vi "SDCP SMF Receiver and Transmitter - Transmit using data fromTx Table.vi"(3 "error in (no error)":errorcluster, 5 "Table Control":refnum<vi>) -> (0 "error out":errorcluster)   [LabVIEW 2020]
uses:
  Typedefs/SDCP SMF Receiver and Transmitter - Transmit Table Element.ctl
  Typedefs/SDCP SMF logger - SMF with timestamp.ctl
panel:
  out "Update table":bool
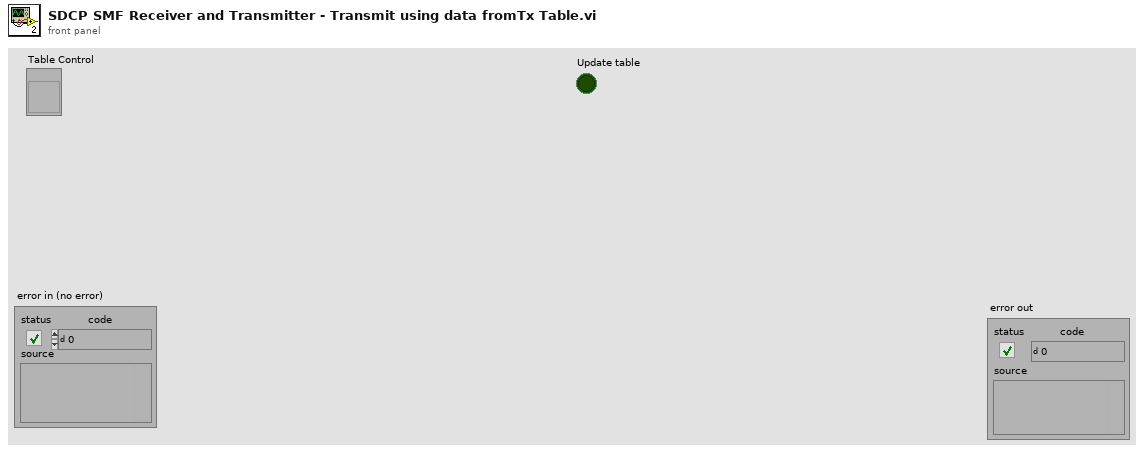
[diagram p1: front panel]
types:
  T1 = typedef "SDCP SMF Receiver and Transmitter - Transmit Table Element.ctl" = cluster{"Frame ID":i32, "Frame Name":string, "Data Bytes":u8[], "Cycle time (ms)":i32, "Counter":i32, "Trigger mode":enum16{"Triggered", "Cyclic"}, "Trigger state":enum16{"Stop cyclic trigger", "Start cyclic trigger", "Stop single trigger", "Start single trigger"}, "Parameter names":string[], "Parameter values":string[]}
  T2 = typedef "SDCP SMF Receiver and Transmitter - Notifier and Queues.ctl" = cluster{"Trace Queue":refnum<queue>, "Tx - Log Table Queue":refnum<queue>, "Tx - User Queue":refnum<queue>, "Rx - Log Table Queue":refnum<queue>, "Rx - User Queue":refnum<queue>, "Log status Notifier":refnum<notifier>, "Plot Queue":refnum<queue>}
  T3 = enum16{"Stop cyclic trigger", "Start cyclic trigger", "Stop single trigger", "Start single trigger"}
  T4 = typedef "SDCP SMF logger - SMF with timestamp.ctl" = cluster{"Bytes":u8[], "Checksum":bool, "Time (ms)":u32, "Tx/Rx":string}
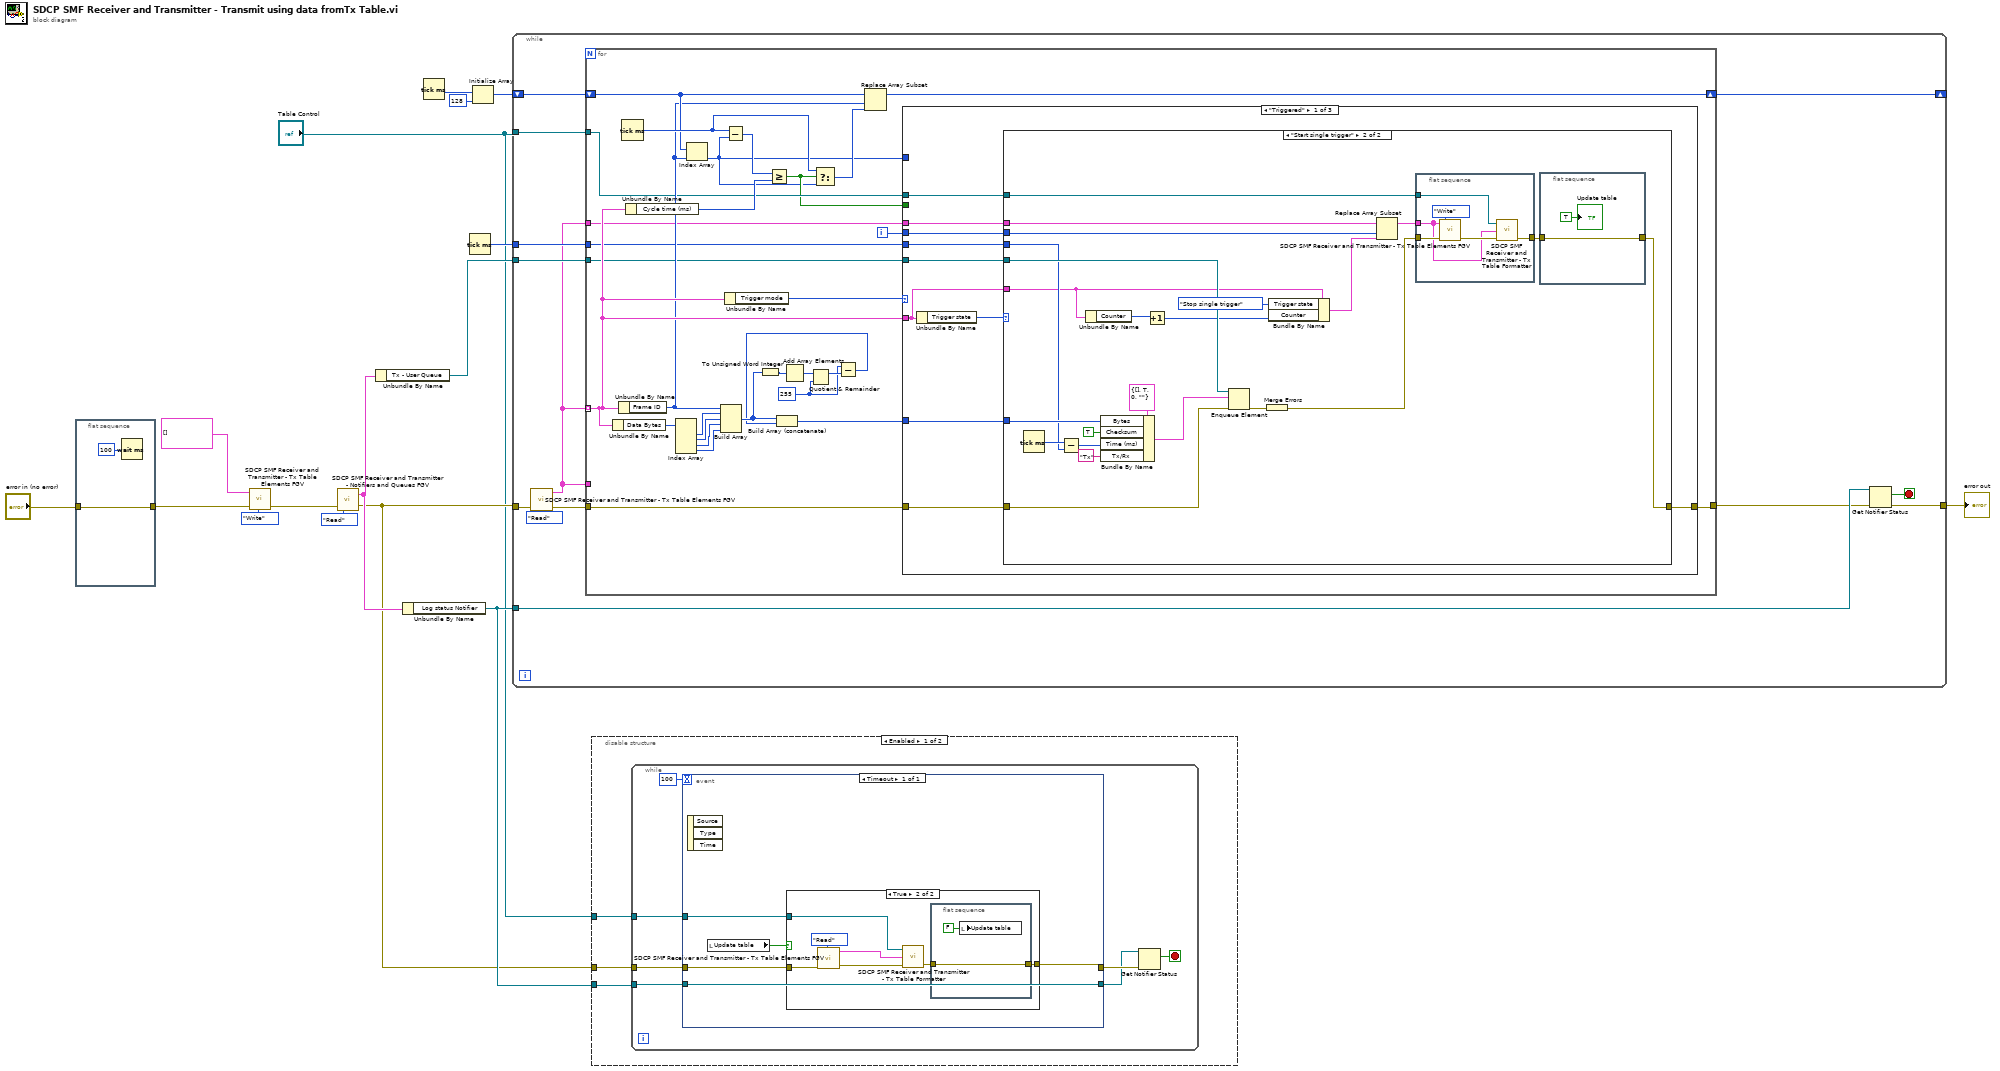
[diagram p0: block diagram]
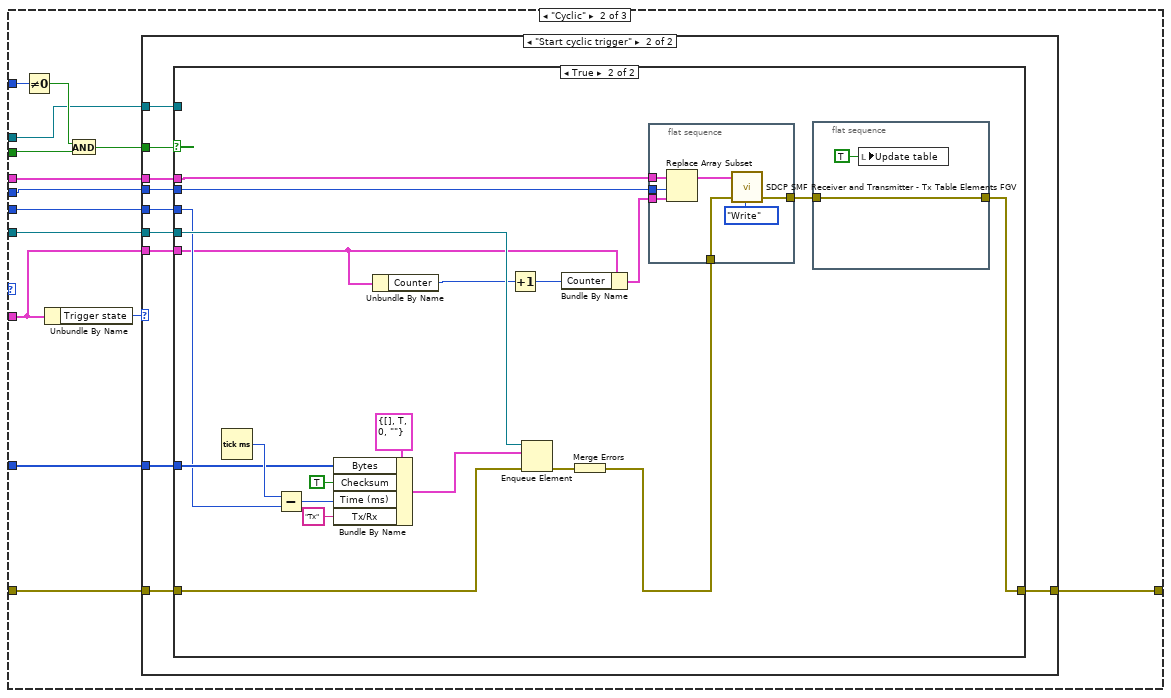
[diagram p5: hidden frame]
diagram:
  n1 = flat-sequence {
    tunnel: "error in (no error)" -> [w18]
    tunnel: [w18] -> w4
    frame #0 {
      n2 = Wait (ms)(milliseconds to wait=u32 100) -> ()  [unwired: 1 out]
    }
  }
  n3 = call "SDCP SMF Receiver and Transmitter - Tx Table Elements FGV.vi"("error in (no error)"=w4, "Command"=enum16{"Read", "Write"}."Write", "Table elements in"=T1[] []) -> ("error out"=w3:errorcluster)  [unwired: 1 in, 1 out]
  n4 = call "SDCP SMF Receiver and Transmitter - Notifiers and Queues FGV.vi"("error in (no error)"=w3, "Command"=enum16{"Initialize", "Read", "Deinitialize"}."Read") -> ("error out"=w7:errorcluster, "Output"=w14:T2)
  n5 = Unbundle By Name(w14) -> ("Tx - User Queue"=w15:refnum<queue>)
  n6 = Unbundle By Name(w14) -> ("Log status Notifier"=w8:refnum<notifier>)
  n7 = Tick Count (ms)() -> (millisecond timer value=w11:u32)
  n8 = Tick Count (ms)() -> (millisecond timer value=w9:u32)
  n9 = Initialize Array(w11, 128 ("dimension size")) -> (w12:u32[])
  n10 = while {
    tunnel: "Table Control" -> [w19]
    tunnel: [w31] -> w16
    tunnel: w7 -> [w28]
    tunnel: w15 -> [w21]
    tunnel: w8 -> [w30]
    shift-right: [w23] -> _
    shift-left: w12 -> [w24]
    tunnel: w9 -> [w22]
    stop <- w29 stop-if-true
    n11 = call "SDCP SMF Receiver and Transmitter - Tx Table Elements FGV.vi"("error in (no error)"=w28, "Command"=enum16{"Read", "Write"}."Read") -> ("error out"=w25:errorcluster, "Table elements out"=w20:T1[])  [unwired: 2 in]
    n12 = for {
      tunnel: [w55] -> w26
      tunnel: w25 -> [w53]
      tunnel: w20 -> [w52] mode=indexing
      shift-right: [w56] -> w23
      shift-left: w24 -> [w58]
      tunnel: w20 -> [_]
      tunnel: w22 -> [w38]
      tunnel: w21 -> [w37]
      tunnel: w20 -> [w36]
      tunnel: w19 -> [w34]
      i -> [w35]
      w42 = u16 255 ("y")
      n13 = Unbundle By Name(w52) -> ("Data Bytes"=w51:u8[])
      n14 = Unbundle By Name(w52) -> ("Frame ID"=w50:i32)
      n15 = Tick Count (ms)() -> (millisecond timer value=w59:u32)
      n16 = Unbundle By Name(w52) -> ("Cycle time (ms)"=w60:i32)
      n17 = Index Array(array=w51) -> (element #1=w49:u8, element #2=w48:u8, element #3=w47:u8, element #4=w46:u8)  [unwired: 4 in]
      n18 = Index Array(array=w58, index=w50) -> (element=w32:u32)
      n19 = Build Array(w50, w49, w48, w47, w46) -> (w41:i32[])
      n20 = Unbundle By Name(w52) -> ("Trigger mode"=w54:enum16{"Triggered", "Cyclic"})
      n21 = Subtract(x=w59, y=w32) -> (x-y=w61:u32)
      n22 = To Unsigned Word Integer(number=w41) -> (unsigned 16bit integer=w45:u16[])
      n23 = Greater Or Equal?(x=w61, y=w60) -> (x >= y?=w33:bool)
      n24 = Add Array Elements(numeric array=w45) -> (sum=w44:u16)
      n25 = Quotient & Remainder(x=w44, y=w42) -> (x-y*floor(x/y)=w43:u16)  [unwired: 1 out]
      n26 = Select(t=w59, s=w33, f=w32) -> (s? t:f=w57:u32)
      n27 = Subtract(x=w42, y=w43) -> (x-y=w40:u16)
      n28 = Build Array (concatenate)(w41, w40) -> (w39:i32[])
      n29 = Replace Array Subset(array=w58, new element=w57, index=w50) -> (w56:u32[])
      n30 = case shown="\"Triggered\"" w54 {
        tunnel: w53 -> [w70 w117 w159]
        tunnel: [w69 w111 w159] -> w55
        tunnel: w52 -> [w64 w107 _]
        tunnel: w39 -> [w68 w110 _]
        tunnel: w38 -> [w67 w108 _]
        tunnel: w37 -> [w66 w109 _]
        tunnel: w36 -> [w65 w106 _]
        tunnel: w35 -> [w63 w105 _]
        tunnel: w34 -> [w62 w104 _]
        tunnel: w33 -> [_ w115 _]
        tunnel: w32 -> [_ w113 _]
        frame "Triggered" {
          n31 = Unbundle By Name(w64) -> ("Trigger state"=w71:T3)
          n32 = case shown="\"Start single trigger\"" w71 {
            tunnel: w70 -> [w72 w91]
            tunnel: [w72 w73] -> w69
            tunnel: w68 -> [_ w93]
            tunnel: w67 -> [_ w87]
            tunnel: w66 -> [_ w95]
            tunnel: w65 -> [_ w84]
            tunnel: w64 -> [_ w77]
            tunnel: w63 -> [_ w81]
            tunnel: w62 -> [_ w79]
            frame "Stop single trigger", Default {
            }
            frame "Start single trigger" {
              n33 = Tick Count (ms)() -> (millisecond timer value=w88:u32)
              n34 = Subtract(x=w88, y=w87) -> (x-y=w86:u32)
              n35 = Unbundle By Name(w77) -> ("Counter"=w76:i32)
              n36 = Bundle By Name(cluster=T4 {"Bytes"=[], "Checksum"=TRUE, "Time (ms)"=0, "Tx/Rx"=""} ("element"), "Bytes"=w93, "Checksum"=TRUE, "Time (ms)"=w86, "Tx/Rx"="Tx") -> (w89:T4)
              n37 = Increment(x=w76) -> (x+1=w75:i32)
              n38 = Enqueue Element(queue=w95, element=w89, error in (no error)=w91) -> (error out=w90:errorcluster)  [unwired: 1 in, 2 out]
              n39 = Merge Errors(w90) -> (w80:errorcluster)
              n40 = Bundle By Name(cluster=w77, "Trigger state"=T3."Stop single trigger", "Counter"=w75) -> (w82:T1)
              n41 = Replace Array Subset(array=w84, new element=w82, index=w81) -> (w78:T1[])
              n42 = flat-sequence {
                tunnel: w80 -> [w102]
                tunnel: [w100] -> w74
                tunnel: w79 -> [w99]
                tunnel: w78 -> [w98]
                frame #0 {
                  n43 = call "SDCP SMF Receiver and Transmitter - Tx Table Elements FGV.vi"("error in (no error)"=w102, "Command"=enum16{"Read", "Write"}."Write", "Table elements in"=w98) -> ("error out"=w101:errorcluster)  [unwired: 1 in, 1 out]
                  n44 = call "SDCP SMF Receiver and Transmitter - Tx Table Formatter.vi"("error in (no error)"=w101, "Transmit table elements"=w98, "Table Control"=w99) -> ("error out"=w100:errorcluster)  [unwired: 2 in]
                }
              }
              n45 = flat-sequence {
                tunnel: w74 -> [w97]
                tunnel: [w97] -> w73
                frame #0 {
                  "Update table" <- TRUE ("Update table")
                }
              }
            }
          }
        }
        frame "Cyclic" {
          n46 = Not Equal To 0?(x=w113) -> (x != 0?=w114:bool)
          n47 = Unbundle By Name(w107) -> ("Trigger state"=w116:T3)
          n48 = And(x=w114, y=w115) -> (x .and. y?=w112:bool)
          n49 = case shown="\"Start cyclic trigger\"" w116 {
            tunnel: w117 -> [w118 w128]
            tunnel: w112 -> [_ w126]
            tunnel: [w118 w127] -> w111
            tunnel: w110 -> [_ w125]
            tunnel: w109 -> [_ w124]
            tunnel: w108 -> [_ w123]
            tunnel: w107 -> [_ w122]
            tunnel: w106 -> [_ w121]
            tunnel: w105 -> [_ w120]
            tunnel: w104 -> [_ w119]
            frame "Stop cyclic trigger", Default {
            }
            frame "Start cyclic trigger" {
              n50 = case shown="True" w126 {
                tunnel: w128 -> [w129 w141]
                tunnel: [w129 w130] -> w127
                tunnel: w125 -> [_ w142]
                tunnel: w124 -> [_ w140]
                tunnel: w123 -> [_ w139]
                tunnel: w122 -> [_ w138]
                tunnel: w121 -> [_ w135]
                tunnel: w120 -> [_ w134]
                tunnel: w119 -> [_ _]
                frame False {
                }
                frame True {
                  n51 = Tick Count (ms)() -> (millisecond timer value=w145:u32)
                  n52 = Subtract(x=w145, y=w139) -> (x-y=w144:u32)
                  n53 = Bundle By Name(cluster=T4 {"Bytes"=[], "Checksum"=TRUE, "Time (ms)"=0, "Tx/Rx"=""} ("element"), "Bytes"=w142, "Checksum"=TRUE, "Time (ms)"=w144, "Tx/Rx"="Tx") -> (w146:T4)
                  n54 = Unbundle By Name(w138) -> ("Counter"=w136:i32)
                  n55 = Increment(x=w136) -> (x+1=w137:i32)
                  n56 = Enqueue Element(queue=w140, element=w146, error in (no error)=w141) -> (error out=w147:errorcluster)  [unwired: 1 in, 2 out]
                  n57 = Bundle By Name(cluster=w138, "Counter"=w137) -> (w133:T1)
                  n58 = Merge Errors(w147) -> (w132:errorcluster)
                  n59 = flat-sequence {
                    tunnel: w135 -> [w157]
                    tunnel: w134 -> [w156]
                    tunnel: w133 -> [w155]
                    tunnel: w132 -> [w153]
                    tunnel: [w152] -> w131
                    frame #0 {
                      n60 = Replace Array Subset(array=w157, new element=w155, index=w156) -> (w154:T1[])
                      n61 = call "SDCP SMF Receiver and Transmitter - Tx Table Elements FGV.vi"("error in (no error)"=w153, "Command"=enum16{"Read", "Write"}."Write", "Table elements in"=w154) -> ("error out"=w152:errorcluster)  [unwired: 1 in, 1 out]
                    }
                  }
                  n62 = flat-sequence {
                    tunnel: w131 -> [w151]
                    tunnel: [w151] -> w130
                    frame #0 {
                      n63 = local write "Update table"(TRUE ("Update table")) -> ()
                    }
                  }
                }
              }
            }
          }
        }
        frame Default {
        }
      }
    }
    n64 = Get Notifier Status(notifier=w30, error in (no error)=w26) -> (current notification=w29:bool, error out=w31:errorcluster)  [unwired: 3 out]
  }
  "error out" <- w16
  n65 = disable-structure shown="Enabled" {
    disable-tunnel: w8 -> [w162 _]
    disable-tunnel: w7 -> [w161 _]
    disable-tunnel: "Table Control" -> [w160 _]
    frame Enabled {
      n66 = while {
        tunnel: w162 -> [w169]
        tunnel: w161 -> [w168]
        tunnel: w160 -> [w163]
        stop <- w165 stop-if-true
        n67 = event shown="[0] Timeout" {
          selector: _ -> [_]
          dyn-events: _ -> [_]
          timeout: 100 -> [_]
          tunnel: w169 -> [w174]
          tunnel: w168 -> [w173]
          tunnel: [w174] -> w166
          tunnel: [w172] -> w167
          tunnel: w163 -> [w171]
          event Timeout {
            n68 = event-data() -> ()  [unwired: 1 in, 3 out]
            n69 = local read "Update table"() -> (w170:bool)
            n70 = case shown="True" w170 {
              tunnel: w173 -> [w175 w181]
              tunnel: [w175 w176] -> w172
              tunnel: w171 -> [_ w178]
              frame False {
              }
              frame True {
                n71 = call "SDCP SMF Receiver and Transmitter - Tx Table Elements FGV.vi"("error in (no error)"=w181, "Command"=enum16{"Read", "Write"}."Read") -> ("error out"=w180:errorcluster, "Table elements out"=w179:T1[])  [unwired: 2 in]
                n72 = call "SDCP SMF Receiver and Transmitter - Tx Table Formatter.vi"("error in (no error)"=w180, "Transmit table elements"=w179, "Table Control"=w178) -> ("error out"=w177:errorcluster)  [unwired: 2 in]
                n73 = flat-sequence {
                  tunnel: w177 -> [w184]
                  tunnel: [w184] -> w176
                  frame #0 {
                    n74 = local write "Update table"(FALSE ("Update table")) -> ()
                  }
                }
              }
            }
          }
        }
        n75 = Get Notifier Status(notifier=w166, error in (no error)=w167) -> (current notification=w165:bool)  [unwired: 4 out]
      }
    }
    frame Disabled {
    }
  }
